vi "Read (Multiple Responses).vi"(8 "error in (no error)":errorcluster, 9 "Wait Time Between Responses (3)":u32=3, 11 "VISA resource name":refnum<visa-resource-name>) -> (0 "error out":errorcluster, 1 "Response Bundle Array":T2(array[cluster]), 2 "Response String Array":string[](array[string]), 3 "VISA resource name out":refnum<visa-resource-name>, 4 "First Response Bundle":T1, 5 "Number of Replies":i32)   [LabVIEW 2018, in "Zaber A Series.lvlib"]
doc: "Reads all available responses from the Serial buffer. An array containing the complete strings of the responses is returned on the Response String Array output, and the details of the format of the response are described here: http://www.zaber.com/wiki/Manuals/ASCII_Protocol_Manual#Replies. This VI also parses the strings, bundles the components, and returns them as an array of bundles on the Response Bundle Array pin. Additionally a pin returns the number of responses received. \n\nThis VI requires that the Initialize VI has been called with the same serial port."
uses:
  Zaber A Series.lvlib
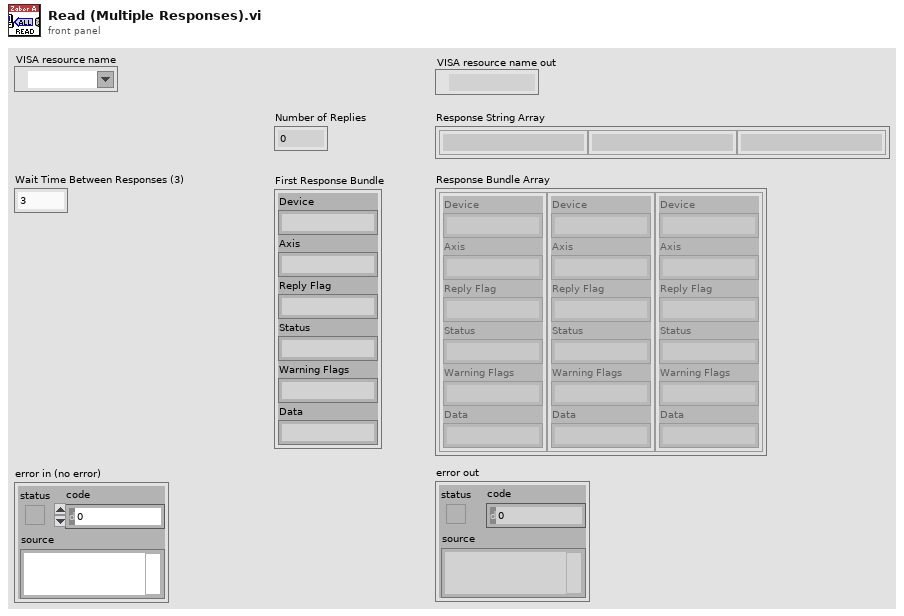
[diagram p1: front panel]
types:
  T1 = cluster{"Device":string, "Axis":string, "Reply Flag":string, "Status":string, "Warning Flags":string, "Data":string}
  T2 = cluster{"Device":string, "Axis":string, "Reply Flag":string, "Status":string, "Warning Flags":string, "Data":string}[]
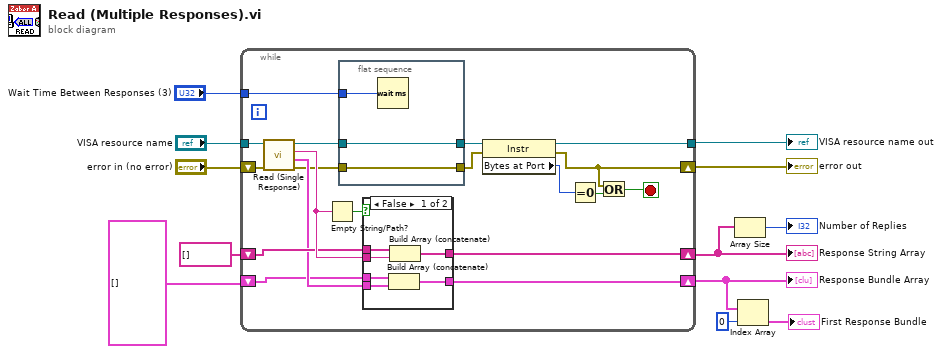
[diagram p0: block diagram]
diagram:
  n1 = while {
    tunnel: "VISA resource name" -> [w31]
    tunnel: [w28] -> w12
    shift-right: [w25] -> w5
    shift-left: string[] [] -> [w24]
    shift-right: [w22] -> w3
    shift-left: T2 [] -> [w21]
    tunnel: "Wait Time Between Responses (3)" -> [w18]
    shift-right: [w13] -> w11
    shift-left: "error in (no error)" -> [w30]
    stop <- w14 stop-if-true
    n2 = call "Read (Single Response).vi"("error in (no error)"=w30, "VISA resource name"=w31) -> ("error out"=w17:errorcluster, "Response Bundle"=w23:T1, "Response"=w26:string, "VISA resource name out"=w20:refnum<visa-resource-name>)  [unwired: 6 in]
    n3 = Empty String/Path?(string/path=w26) -> (empty?=w27:bool)
    n4 = flat-sequence {
      tunnel: w20 -> [w34]
      tunnel: [w34] -> w19
      tunnel: w18 -> [w33]
      tunnel: w17 -> [w32]
      tunnel: [w32] -> w16
      frame #0 {
        n5 = Wait (ms)(milliseconds to wait=w33) -> ()  [unwired: 1 out]
      }
    }
    n6 = case shown="False" w27 {
      tunnel: w26 -> [w40 _]
      tunnel: [w39 w42] -> w25
      tunnel: w24 -> [w38 w42]
      tunnel: w23 -> [w37 _]
      tunnel: [w36 w41] -> w22
      tunnel: w21 -> [w35 w41]
      frame False {
        n7 = Build Array (concatenate)(w35, w37) -> (w36:T2)
        n8 = Build Array (concatenate)(w38, w40) -> (w39:string[])
      }
      frame True {
      }
    }
    n9 = property class="Instr"(reference=w19, error in=w16) -> (reference out=w28:refnum<visa-resource-name>, error out=w13:errorcluster, "Bytes at Port"=w29:u32)
    n10 = Equal To 0?(x=w29) -> (x = 0?=w15:bool)
    n11 = Or(x=w13, y=w15) -> (x .or. y?=w14:bool)
  }
  "VISA resource name out" <- w12
  "error out" <- w11
  "Response String Array" <- w5
  "Response Bundle Array" <- w3
  n12 = Array Size(array=w5) -> (size(s)=→"Number of Replies":i32)
  n13 = Index Array(array=w3, index=0) -> (element=→"First Response Bundle":T1)
